vi "Corr Transducers to Meas Header.vi"(8 "error in":errorcluster, 10 "measurement root path":path, 11 "transducers in":cluster{"channels":T1[], "last path":path} {"channels"."Phase index" min=1 step=1}) -> (0 "error out":errorcluster, 2 "info data out":string, 3 "transducers out":cluster{"channels":T1[], "last path":path} {"channels"."Phase index" min=1 step=1})   [LabVIEW 2018]
doc: "This VI will copy all transducer corrections to the measurement root path."
uses:
  Corr Tranducer Item.ctl
  octave/infolib.lvlibp/Private/Add matrix polymorph parts/2D I64.vi
  octave/infolib.lvlibp/Private/Add matrix polymorph parts/1D String.vi
  octave/infolib.lvlibp/Private/Add matrix polymorph parts/1D I64.vi
  octave/infolib.lvlibp
panel:
  # "ADC:"
  # "ADC:"
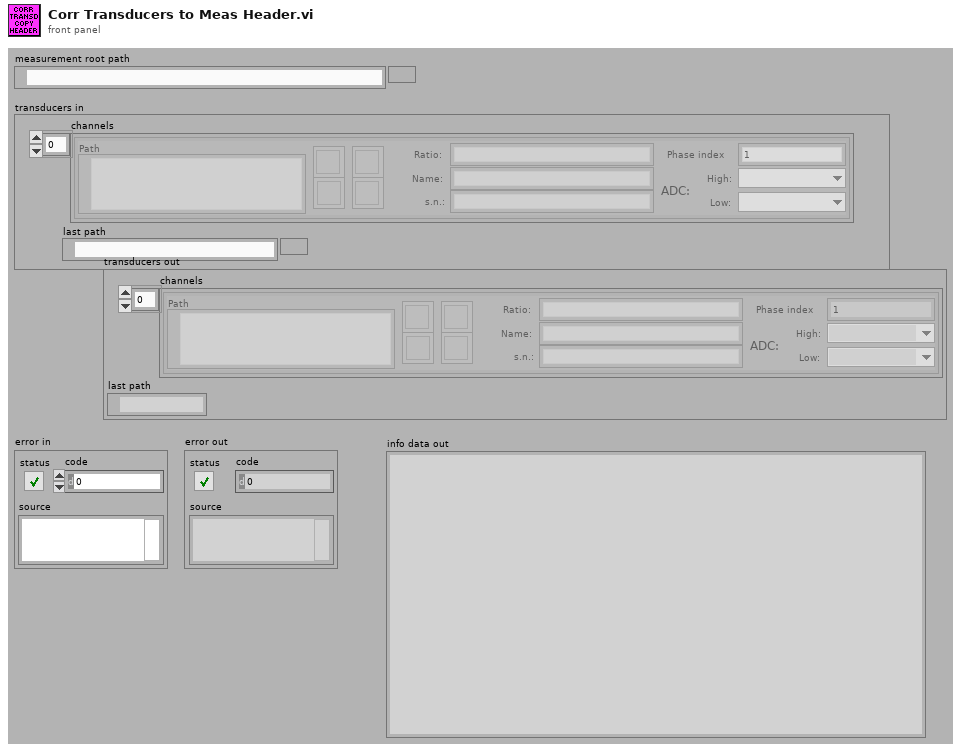
[diagram p1: front panel]
types:
  T1 = typedef "Corr Tranducer Item.ctl" = cluster{"Path":path, "Ratio:":string, "Name:":string, "btn rem":bool, "btn up":bool, "btn down":bool, "s.n.:":string, "btn open":bool, "ratio o/i":dbl, "chn hi":u16, "chn lo":u16, "Phase index":i32}
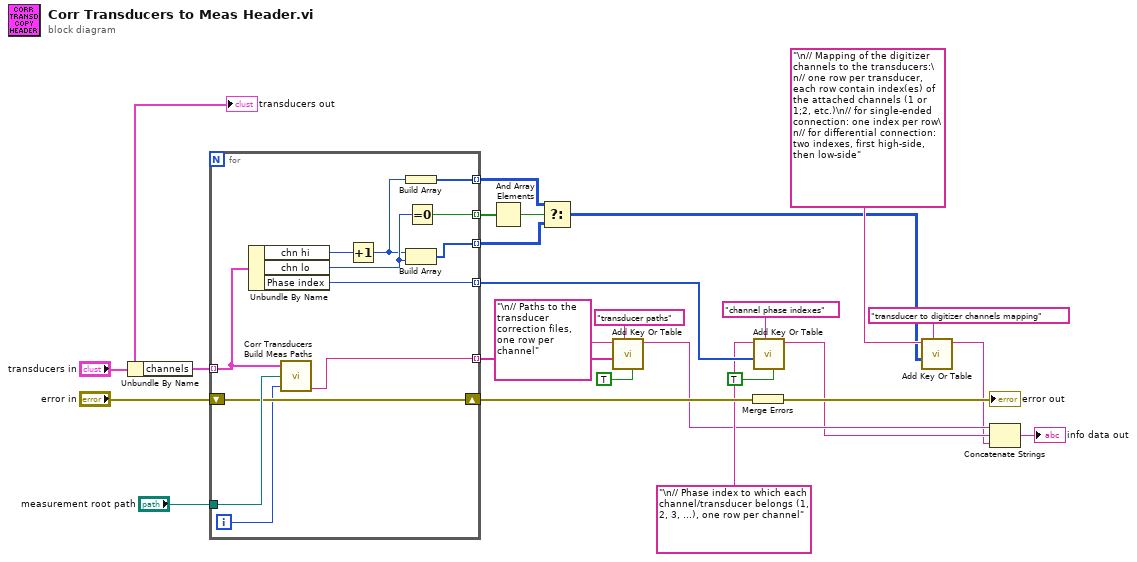
[diagram p0: block diagram]
diagram:
  n1 = Unbundle By Name("transducers in") -> ("channels"=w25:T1[])
  n2 = for {
    tunnel: w25 -> [w34] mode=indexing
    tunnel: "measurement root path" -> [w37]
    shift-right: [w36] -> w23
    shift-left: "error in" -> [w36]
    tunnel: [w35] -> w15 mode=indexing
    tunnel: [w33] -> w17 mode=indexing
    tunnel: [w30] -> w3 mode=indexing
    tunnel: [w28] -> w5 mode=indexing
    tunnel: [w26] -> w2 mode=indexing
    i -> [w31]
    n3 = Unbundle By Name(w34) -> ("chn hi"=w32:u16, "chn lo"=w29:u16, "Phase index"=w33:i32)
    n4 = call "Corr Transducers Build Meas Paths.vi"("transducer"=w34, "measurement folder root path"=w37, "transducer index"=w31) -> ("destination header realtive path"=w35:string)  [unwired: 3 out]
    n5 = Increment(x=w32) -> (x+1=w27:u16)
    n6 = Build Array(w27) -> (w26:u16[])
    n7 = Build Array(w27, w29) -> (w30:u16[])
    n8 = Equal To 0?(x=w29) -> (x = 0?=w28:bool)
  }
  n9 = And Array Elements(Boolean array=w5) -> (logical AND=w4:bool)
  n10 = Select(t=w2, s=w4, f=w3) -> (s? t:f=w1:u16[][])
  n11 = call-poly "Add Key Or Table.vi"("column vector (F)"=TRUE, "key description"="transducer paths", "string"=w15, "info data"="\n// Paths to the transducer correction files, one row per channel") -> ("info data out"=w11:string)  [unwired: 6 in, 1 out]
  n12 = Merge Errors(w23) -> (→"error out":errorcluster)
  n13 = call-poly "Add Key Or Table.vi"("column vector (F)"=TRUE, "key description"="channel phase indexes", "numeric"=w17, "info data"="\n// Phase index to which each channel/transducer belongs (1, 2, 3, ...), one row per channel") -> ("info data out"=w10:string)  [unwired: 6 in, 1 out]
  n14 = call-poly "Add Key Or Table.vi"("key description"="transducer to digitizer channels mapping", "numeric"=w1, "info data"="\n// Mapping of the digitizer channels to the transducers:\n// one row per transducer, each row contain index(es) of the attached channels (1 or 1;2, etc.)\n// for single-ended connection: one index per row\n// for differential connection: two indexes, first high-side, then low-side") -> ("info data out"=w9:string)  [unwired: 8 in]
  n15 = Concatenate Strings(w11, w10, w9) -> (→"info data out":string)
  "transducers out" <- "transducers in"
